vi "Creators Is Created Event.vi"(10 "Created Event Alias":string, 11 "Base Event jettl in":refnum<class "Base Event jettl.lvclass">) -> (2 "Is Created Event?":bool, 3 "Base Event jettl out":refnum<class "Base Event jettl.lvclass">)   [LabVIEW 2021, in "jettl.lvlib" / "Base Event jettl.lvlib" / "Base Event jettl.lvclass"]
uses:
  Base Event jettl.lvclass
  Base Event jettl.lvclass/Base Event jettl.ctl
  Queue Mailbox/Queue Mailbox.lvlib
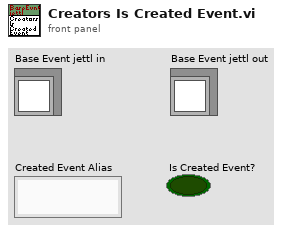
[diagram p1: front panel]
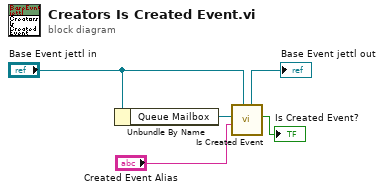
[diagram p0: block diagram]
diagram:
  n1 = Unbundle By Name("Base Event jettl in") -> ("Queue Mailbox"=w3:refnum<data-value>)
  n2 = call "Is Created Event.vi"("jettl in"="Base Event jettl in", "Created Event Alias"="Created Event Alias", "Queue Mailbox"=w3) -> ("Is Created Event?"=→"Is Created Event?":bool, "jettl out"=→"Base Event jettl out":refnum<class "Base Event jettl.lvclass">)  [unwired: 7 in]
